vi "Journalisation.vi"(0 "time string":string, 2 "Data":string, 3 "Booléen":bool, 4 "Entête":string, 5 "Fichier origine":string, 6 "date string":string, 7 "file refnum":refnum<file>) -> (1 "refnum out":refnum<file>)   [LabVIEW 2018]
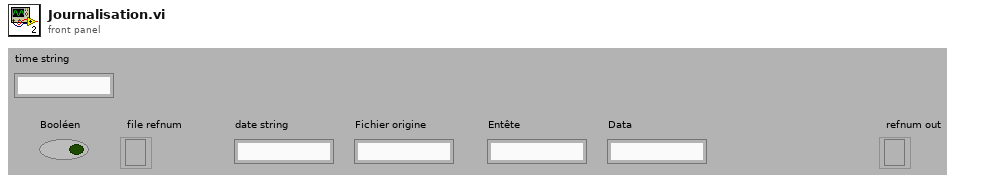
[diagram p1: front panel]
types:
  T1 = enum16{"open", "replace", "create", "open or create", "replace or create", "replace or create with confirmation"}
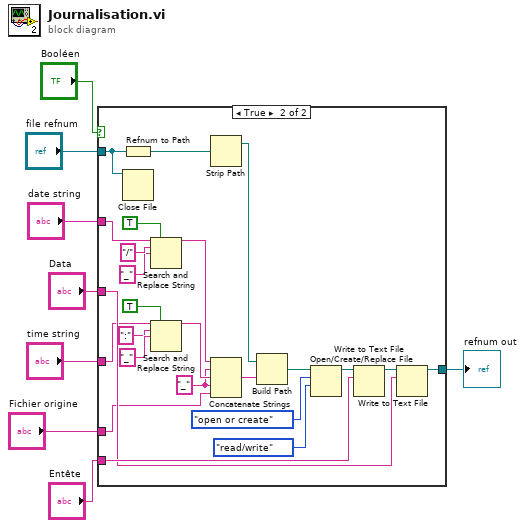
[diagram p0: block diagram]
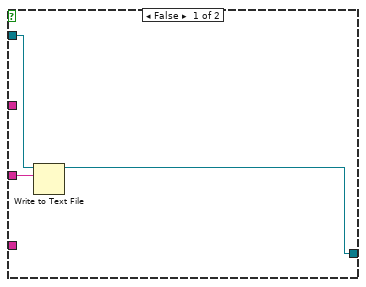
[diagram p2: hidden frame]
diagram:
  n1 = case shown="True" "Booléen" {
    tunnel: "file refnum" -> [w11 w25]
    tunnel: [w10 w35] -> w3
    tunnel: "date string" -> [_ w30]
    tunnel: "Fichier origine" -> [_ w14]
    tunnel: "Entête" -> [_ w23]
    tunnel: "Data" -> [w9 w22]
    tunnel: "time string" -> [_ w15]
    frame False {
      n2 = Write to Text File(file (use dialog)=w11, text=w9) -> (refnum out=w10:refnum<file>)  [unwired: 2 in, 2 out]
    }
    frame True {
      w12 = "_" ("chaîne")
      n3 = Refnum to Path(1:w25) -> (0:w24:path)
      n4 = Close File(refnum=w25) -> ()  [unwired: 1 in, 2 out]
      n5 = Search and Replace String(replace all?=TRUE ("tout remplacer ? (F)"), input string=w30, search string="/" ("chaîne recherchée"), replace string="_" ("chaîne de remplacement (\"\")")) -> (result string=w29:string)  [unwired: 4 in, 3 out]
      n6 = Search and Replace String(replace all?=TRUE ("tout remplacer ? (F)"), input string=w15, search string=":" ("chaîne recherchée"), replace string="_" ("chaîne de remplacement (\"\")")) -> (result string=w13:string)  [unwired: 4 in, 3 out]
      n7 = Strip Path(path=w24) -> (stripped path=w20:path)  [unwired: 1 out]
      n8 = Concatenate Strings(w29, w12, w13, w12, w14) -> (w19:string)
      n9 = Build Path(base path=w20, name or relative path=w19) -> (appended path=w33:path)
      n10 = Open/Create/Replace File(file path (use dialog)=w33, operation (0:open)=T1."open or create" ("opération (0 : open)"), access (0:read/write)=enum16{"read/write", "read-only", "write-only"}."read/write" ("accès (0 : read/write)")) -> (refnum out=w34:refnum<file>)  [unwired: 1 in, 4 out]
      n11 = Write to Text File(file (use dialog)=w34, text=w23) -> (refnum out=w21:refnum<file>)  [unwired: 2 in, 2 out]
      n12 = Write to Text File(file (use dialog)=w21, text=w22) -> (refnum out=w35:refnum<file>)  [unwired: 2 in, 2 out]
    }
  }
  "refnum out" <- w3
